vi "MIC working.vi"() -> ()   [LabVIEW 2022 SP3]
uses:
  <vilib>/DAQmx/read.llb/DAQmx Read (Analog Wfm 1Chan NSamp).vi
  <vilib>/DAQmx/create/channels.llb/DAQmx Create Channel (AI-Sound Pressure-Microphone).vi
  <vilib>/DAQmx/configure/timing.llb/DAQmx Timing (Sample Clock).vi
  <vilib>/DAQmx/miscellaneous.llb/DAQmx Fill In Error Info.vi
panel:
  in  "rate":dbl=1000.0 format="%0.2f"
  in  "input terminal configuration":i32(ring)=-1 items=["default"=-1, "RSE"=10083, "NRSE"=10078, "Differential"=10106, "Pseudodifferential"=12529]
  in  "physical channels":tag
  out "Waveform Chart":waveform(dbl)(graph)
  out "data":dbl format="%0.2f"
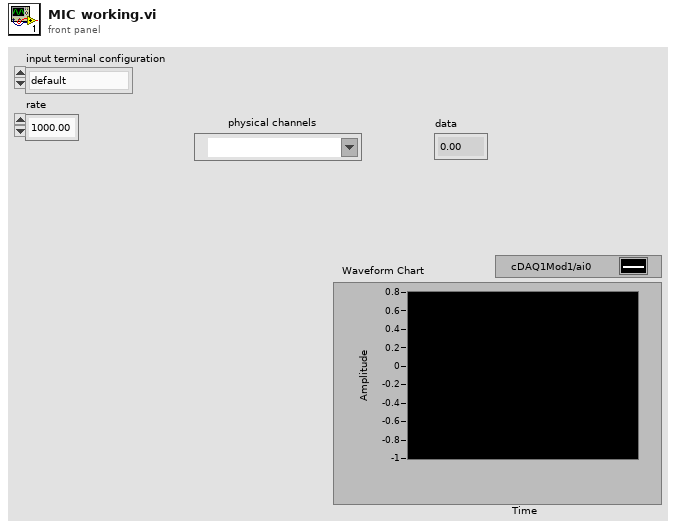
[diagram p1: front panel]
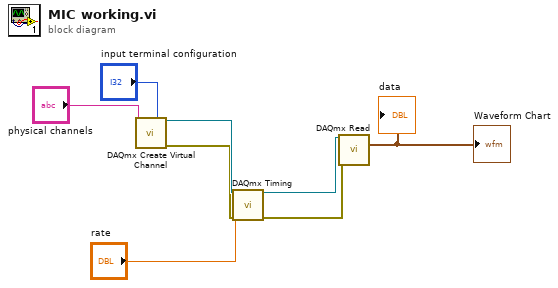
[diagram p0: block diagram]
diagram:
  n1 = call-poly <vilib>:"DAQmx Create Virtual Channel.vi"("input terminal configuration"="input terminal configuration", "physical channels"="physical channels") -> ("task out"=w5:refnum<k21>, "error out"=w4:errorcluster)  [unwired: 12 in]
  n2 = call-poly <vilib>:"DAQmx Timing.vi"("task/channels in"=w5, "rate"="rate", "error in"=w4) -> ("task out"=w3:refnum<k21>, "error out"=w2:errorcluster)  [unwired: 11 in]
  n3 = call-poly <vilib>:"DAQmx Read.vi"("task/channels in"=w3, "error in"=w2) -> ("data"=→"data" →"Waveform Chart":waveform(dbl))  [unwired: 11 in, 2 out]
